vi "Static.vi"() -> ()   [LabVIEW 2020, in "Panel.lvlib" / "Panel Registry.lvclass"]
uses:
  <vilib>/MGI/Panel Manager/Panel/Panel Registry/Panel Registry.lvclass
panel:
  out "Last Event":variant
  out "Panel State":variant
  out "Event Lookup":variant
  out "Parent Lookup":variant
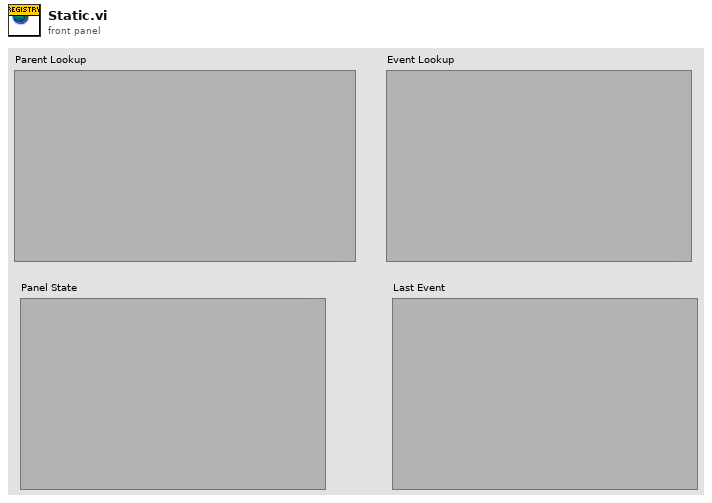
[diagram p1: front panel]
diagram:
